vi "Read CtlRef.vi"(8 "error in (no error)":errorcluster, 11 "TreeItemCloseMsg in":refnum<class "TreeItemCloseMsg.lvclass">) -> (0 "error out":errorcluster, 2 "CtlRef":refnum<vi>, 3 "TreeItemCloseMsg out":refnum<class "TreeItemCloseMsg.lvclass">)   [LabVIEW 2017, in "ActorEvents.lvlib" / "TreeItemCloseMsg.lvclass"]
uses:
  TreeItemCloseMsg.lvclass
  TreeItemCloseMsg.lvclass/TreeItemCloseMsg.ctl
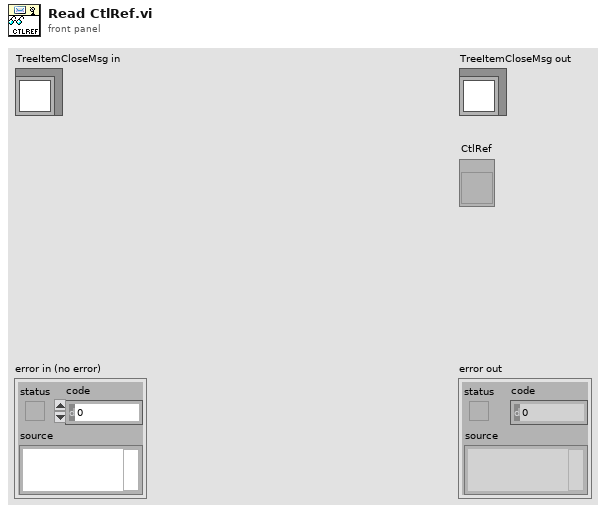
[diagram p1: front panel]
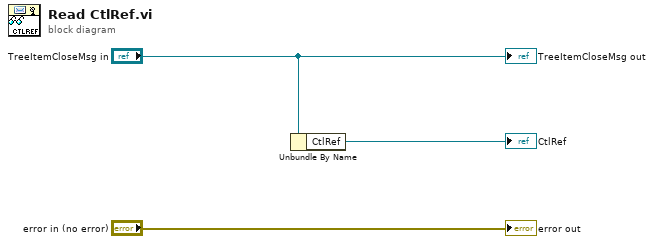
[diagram p0: block diagram]
diagram:
  n1 = Unbundle By Name("TreeItemCloseMsg in") -> ("CtlRef"=→"CtlRef":refnum<vi>)
  "error out" <- "error in (no error)"
  "TreeItemCloseMsg out" <- "TreeItemCloseMsg in"
